vi "Create.vi"(8 "error in (no error)":errorcluster, 9 "Authentication":refnum<class "Authentication.lvclass">, 10 "Policies":refnum<class "Policies.lvclass">, 11 "Credentials":refnum<class "Credentials.lvclass">) -> (0 "error out":errorcluster, 3 "Session out":refnum<class "Session.lvclass">)   [LabVIEW 2016, in "Session.lvclass"]
uses:
  Session.lvclass
  Credentials/Credentials.lvclass
  Policies/Policies.lvclass
  Authentication/Authentication.lvclass
  Session.lvclass/Session.ctl
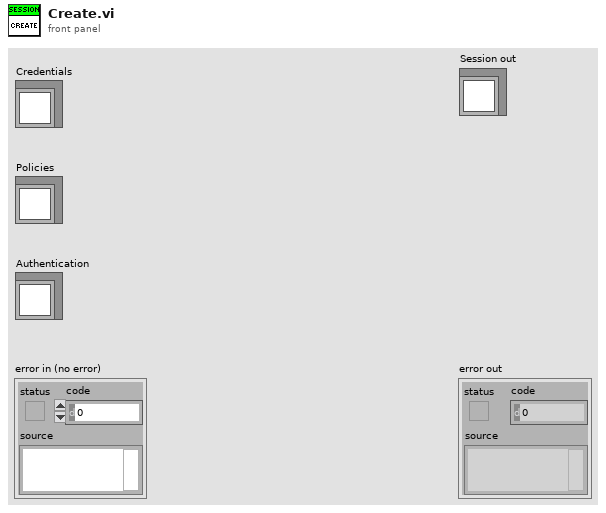
[diagram p1: front panel]
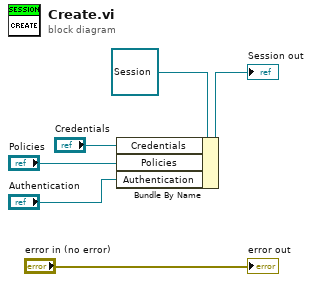
[diagram p0: block diagram]
diagram:
  n1 = Bundle By Name(cluster=refnum<class "Session.lvclass"> refnum ("Session out"), "Credentials"="Credentials", "Policies"="Policies", "Authentication"="Authentication") -> (→"Session out":refnum<class "Session.lvclass">)
  "error out" <- "error in (no error)"
